vi "finalize_lib_tsmaster.vi"(8 "error in (no error)":errorcluster, 11 "Path":path) -> (0 "error out":errorcluster, 3 "Path output":path)   [LabVIEW 2014]
doc: "Function Introduction ：\nRelease TsMasterApi module\nCall location ：\nRelease the resources used by TsMasterApi before exiting the program."
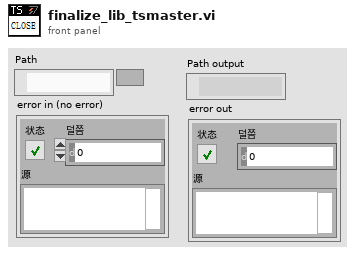
[diagram p1: front panel]
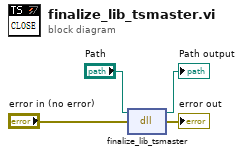
[diagram p0: block diagram]
diagram:
  n1 = dll-call lib="D:/Program Files (x86)/TOSUN/TSMaster/Data/SDK/lib/x86/TSMaster.dll" fn="finalize_lib_tsmaster"(path in="Path", error in="error in (no error)") -> (path out=→"Path output":path, error out=→"error out":errorcluster)  [unwired: 2 in]
